vi "Read Self-Models.vi"(8 "error in (no error)":errorcluster, 11 "MVVM Abstruct Model in":refnum<class "MVVM Abstruct Model.lvclass">) -> (0 "error out":errorcluster, 2 "ActorMap.lvclass":refnum<class "ActorMap.lvclass">, 3 "MVVM Abstruct Model out":refnum<class "MVVM Abstruct Model.lvclass">)   [LabVIEW 2020, in "MMVVM Framework.lvlib" / "MVVM Abstruct Model.lvlib" / "MVVM Abstruct Model.lvclass"]
uses:
  MVVM Abstruct Model.lvclass
  ActorMap/ActorMap.lvclass
  MVVM Abstruct Model.lvclass/MVVM Abstruct Model.ctl
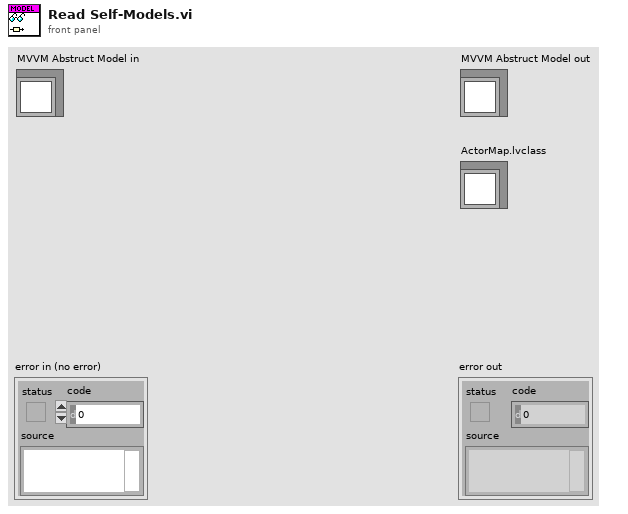
[diagram p1: front panel]
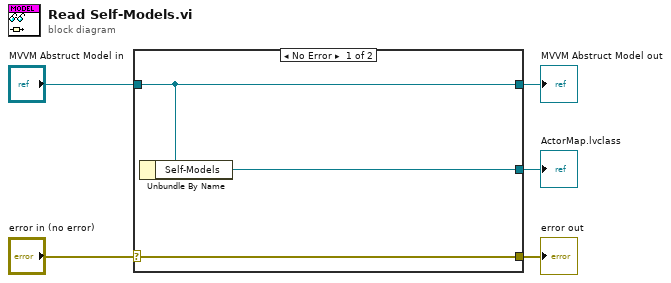
[diagram p0: block diagram]
diagram:
  n1 = case shown="No Error" "error in (no error)" {
    selector: "error in (no error)" -> [w8 w9]
    tunnel: [w8 w9] -> w4
    tunnel: [w7 w10] -> w2
    tunnel: "MVVM Abstruct Model in" -> [w7 w10]
    tunnel: [w6 _] -> w1
    frame No Error {
      n2 = Unbundle By Name(w7) -> ("Self-Models"=w6:refnum<class "ActorMap.lvclass">)
    }
    frame Error {
    }
  }
  "error out" <- w4
  "MVVM Abstruct Model out" <- w2
  "ActorMap.lvclass" <- w1
